vi "advanced_cont_memtest_1channel-v06.vi"(0 "Pulse AI task in":refnum<k21>, 1 "replicates":i32=5, 4 "Pulse AO task in":refnum<k21>, 5 "error in":errorcluster, 7 "memtest":T2={"Samples to Read"=1000, "Rate (Hz)"=20000.0, "Amplitude (mV/pA)"=10.0, "Offset (mV/pA)"=-60.0, "Frequency (Hz)"=-60.0, "duty cycle (%)"=50.0, "phase"=0.0} {"phase" format="%.2p"; "duty cycle (%)" format="%0.2f"}, 11 "which clamp":enum16{"VClamp", "IClamp"}(ring)) -> (9 "Power Spectrum":dbl[](graph), 12 "cell quality bad":bool, 13 "avg peak height":dbl, 14 "Pulse AI task out":refnum<k21>, 15 "data out (pA or mV)":waveform(dbl)[](graph), 16 "cell stats":T1 {"STD" format="%010.2f"; "Variance" format="%010.2f"; "Rt (MOhms)" format="%010.2f"; "tau (ms)" format="%08.2g"; "Cm (pF)" format="%08.2f"; "Ra (MOhms)" format="%010.2f"; "Rm (MOhms)" format="%010.2f"; "Ihold (pA)" format="%010.2f"}, 17 "cont memtest error?":bool, 18 "Pulse AO task out":refnum<k21>, 19 "error out":errorcluster)   [LabVIEW 2019]
uses:
  controls/memtest_def.ctl
  wc_protocol_v1.003 Folder/whole_cell_protocol/Controls/cell_stats-v02.ctl
  <vilib>/DAQmx/read.llb/DAQmx Read (Analog Wfm 1Chan NSamp).vi
  <vilib>/DAQmx/miscellaneous.llb/DAQmx Fill In Error Info.vi
  <resource>/objmgr/daqmx.rc
panel:
  out "AvailSampPerChan":u32
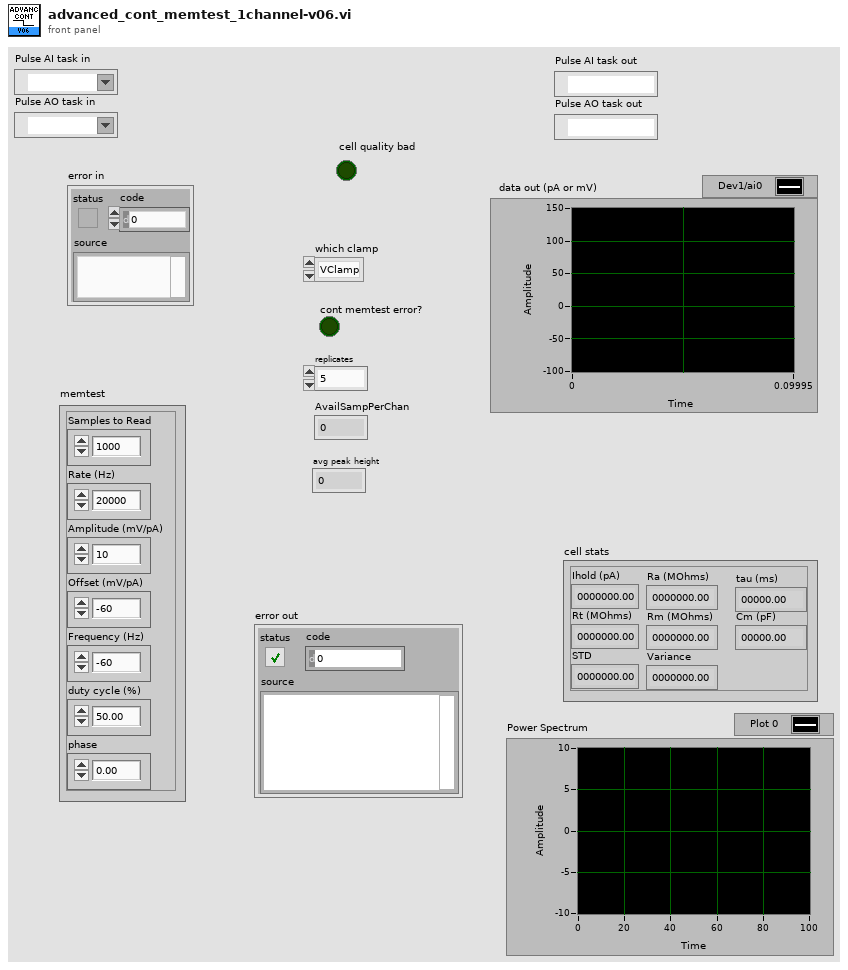
[diagram p1: front panel]
types:
  T1 = typedef "cell_stats-v02.ctl" = cluster{"Ihold (pA)":dbl, "Rm (MOhms)":dbl, "Ra (MOhms)":dbl, "Cm (pF)":dbl, "tau (ms)":dbl, "Rt (MOhms)":dbl, "Variance":dbl, "STD":dbl}
  T2 = typedef "memtest_def.ctl" = cluster{"Samples to Read":i32, "Rate (Hz)":dbl, "Amplitude (mV/pA)":dbl, "Offset (mV/pA)":dbl, "Frequency (Hz)":dbl, "duty cycle (%)":dbl, "phase":dbl}
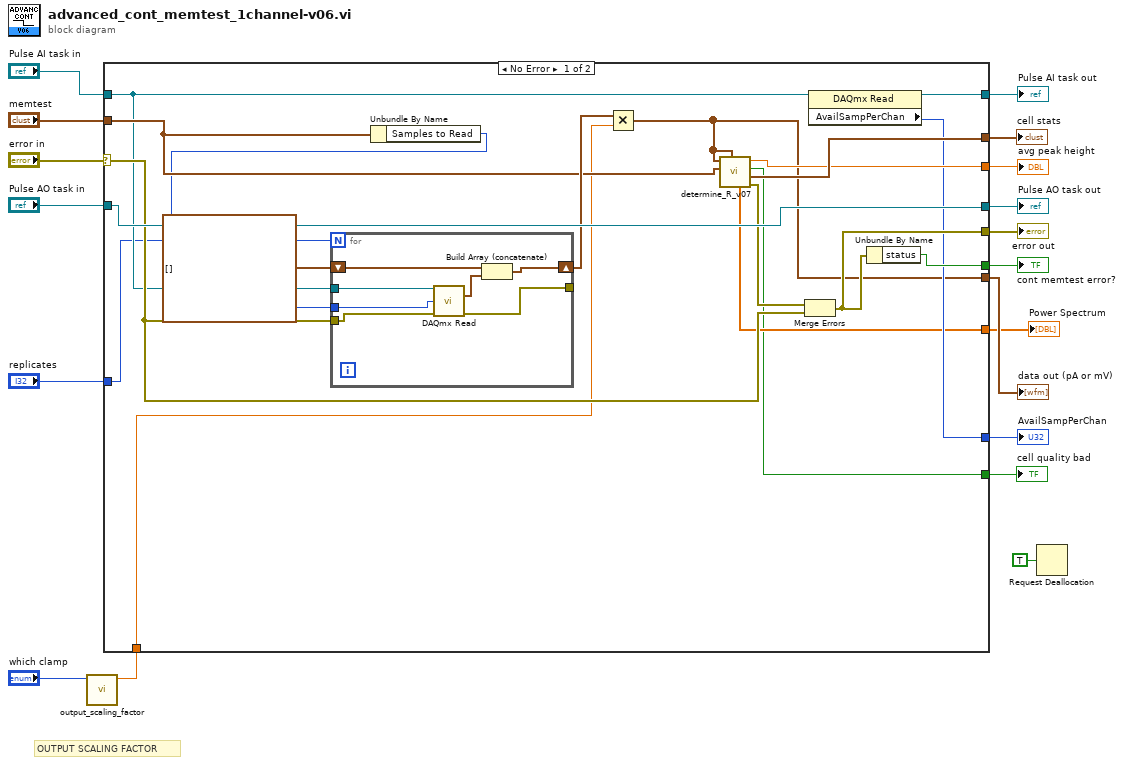
[diagram p0: block diagram]
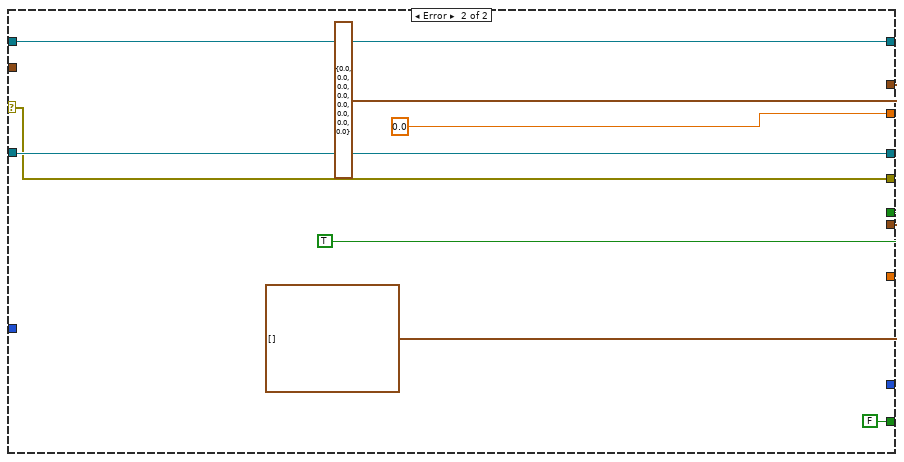
[diagram p2: hidden frame]
diagram:
  # "OUTPUT SCALING FACTOR"
  n1 = call "output_scaling_factor.vi"("which clamp"="which clamp") -> ("output scaling factor"=w11:dbl)  [unwired: 10 in]
  n2 = case shown="No Error" "error in" {
    selector: "error in" -> [w32 w49]
    tunnel: "Pulse AI task in" -> [w27 w51]
    tunnel: "Pulse AO task in" -> [w37 w50]
    tunnel: [w33 TRUE ("status")] -> w15
    tunnel: [w37 w50] -> w14
    tunnel: [w36 w51] -> w13
    tunnel: [w34 w49] -> w12
    tunnel: w11 -> [w25 _]
    tunnel: [w29 0.0 ("avg peak height")] -> w8
    tunnel: [w30 T1 {"Ihold (pA)"=0.0, "Rm (MOhms)"=0.0, "Ra (MOhms)"=0.0, "Cm (pF)"=0.0, "tau (ms)"=0.0, "Rt (MOhms)"=0.0, "Variance"=0.0, "STD"=0.0} ("cell stats")] -> w9
    tunnel: "replicates" -> [w22 _]
    tunnel: "memtest" -> [w28 _]
    tunnel: [w20 waveform(dbl)[] []] -> w5
    tunnel: [w26 _] -> w4
    tunnel: [w21 _] -> w3
    tunnel: [w19 FALSE ("cell quality bad")] -> w1
    frame No Error {
      n3 = Unbundle By Name(w28) -> ("Samples to Read"=w23:i32)
      n4 = for {
        N: w22 -> [_]
        tunnel: w27 -> [w44]
        tunnel: w23 -> [w43]
        tunnel: w32 -> [w42]
        tunnel: [w38] -> _
        shift-right: [w41] -> w31
        shift-left: waveform(dbl)[] [] -> [w40]
        n5 = call-poly <vilib>:"DAQmx Read.vi"("task/channels in"=w44, "number of samples per channel"=w43, "error in"=w42) -> ("data"=w39:waveform(dbl), "error out"=w38:errorcluster)  [unwired: 10 in, 1 out]
        n6 = Build Array (concatenate)(w40, w39) -> (w41:waveform(dbl)[])
      }
      n7 = Multiply(x=w31, y=w25) -> (x*y=w20:waveform(dbl)[])
      n8 = call "determine_R_v07.vi"("Pulse Data in (pA)"=w20, "memtest"=w28, "Noise Data in (pA)"=w20) -> ("Power Spectrum"=w21:dbl[], "avg peak height"=w29:dbl, "cell quality bad"=w19:bool, "cell stats"=w30:T1, "error out"=w35:errorcluster)  [unwired: 3 in]
      n9 = Merge Errors(w35, w32) -> (w34:errorcluster)
      n10 = property class="DAQmx Read"(reference=w27) -> (reference out=w36:refnum<k21>, "AvailSampPerChan"=w26:u32)  [unwired: 1 in, 1 out]
      n11 = Unbundle By Name(w34) -> ("status"=w33:bool)
    }
    frame Error {
    }
  }
  "Pulse AI task out" <- w13
  "Pulse AO task out" <- w14
  "cont memtest error?" <- w15
  "error out" <- w12
  "cell stats" <- w9
  "avg peak height" <- w8
  "data out (pA or mV)" <- w5
  "AvailSampPerChan" <- w4
  "Power Spectrum" <- w3
  "cell quality bad" <- w1
  n12 = Request Deallocation(TRUE ("flag")) -> ()
